vi "Create Base to Relative Frame Velocity Transform Matrix.vi"(9 "relative frame angle (rad)":dbl, 10 "y relative position":dbl, 11 "x relative position":dbl) -> (3 "base to relative velocity transform":T1)   [LabVIEW 2017, in "NI_Robotics_Steering Utilities.lvlib"]
doc: "Constructs a transform matrix R to convert from the base frame velocity to the relative frame velocity:\n\nx' = R*x\nx: base frame velocity\nx': relative frame velocity"
uses:
  <vilib>/robotics/Steering/Utilities/NI_Robotics_Steering Utilities.lvlib
  <vilib>/Analysis/Matrix/Datatypes/RealMatrix.ctl
  <vilib>/Analysis/Matrix/NI_Matrix.lvlib
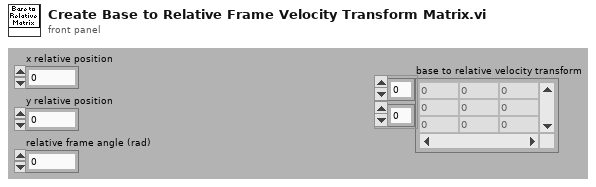
[diagram p1: front panel]
types:
  T1 = typedef "NI_Matrix.lvlib/RealMatrix.ctl" = dbl[][]
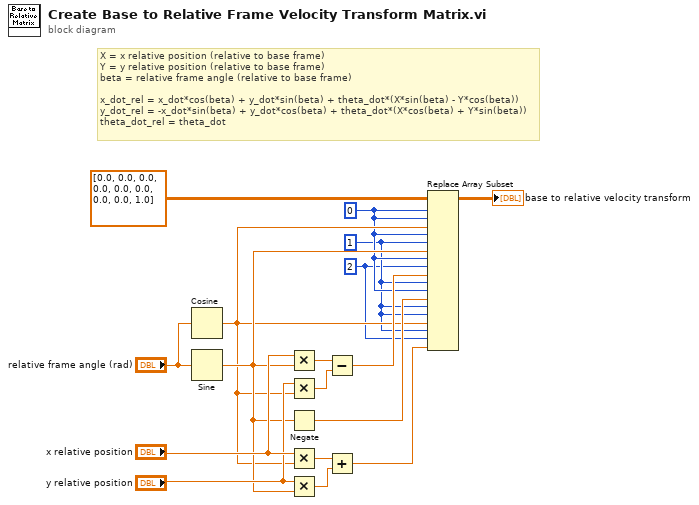
[diagram p0: block diagram]
diagram:
  w2 = 2 ("disabled index (col)")
  w3 = 1 ("disabled index (col)")
  w4 = 0 ("index (row)")
  # "X = x relative position (relative to base frame)\nY = y relative position (relative to base frame)\nbeta = relative frame angle (relative to base frame)\n\nx_dot_rel = x_dot*cos(beta) + y_dot*sin(beta) + theta_dot*(X*sin(beta) - Y*cos(beta))\ny_dot_rel = -x_dot*sin(beta) + y_dot*cos(beta) + theta_dot*(X*cos(beta) + Y*sin(beta))\ntheta_dot_rel = theta_dot"
  n1 = Cosine(x="relative frame angle (rad)") -> (cos(x)=w6:dbl)
  n2 = Sine(x="relative frame angle (rad)") -> (sin(x)=w9:dbl)
  n3 = Multiply(x="x relative position", y=w9) -> (x*y=w11:dbl)
  n4 = Multiply(x="y relative position", y=w6) -> (x*y=w12:dbl)
  n5 = Negate(x=w9) -> (-x=w7:dbl)
  n6 = Multiply(x="x relative position", y=w6) -> (x*y=w13:dbl)
  n7 = Multiply(x="y relative position", y=w9) -> (x*y=w14:dbl)
  n8 = Subtract(x=w11, y=w12) -> (x-y=w8:dbl)
  n9 = Add(x=w13, y=w14) -> (x+y=w5:dbl)
  n10 = Replace Array Subset(array=T1 [[0.0, 0.0, 0.0], [0.0, 0.0, 0.0], [0.0, 0.0, 1.0]] ("appended array"), new element #1=w6, index (row) #1=w4, index (col) #1=w4, new element #2=w9, index (row) #2=w4, index (col) #2=w3, new element #3=w8, index (row) #3=w4, index (col) #3=w2, new element #4=w7, index (row) #4=w3, index (col) #4=w4, new element #5=w6, index (row) #5=w3, index (col) #5=w3, new element #6=w5, index (row) #6=w3, index (col) #6=w2) -> (→"base to relative velocity transform":T1)
